vi "Populate Tree Control Recursive Priv.vi"(4 "Show IDs (True)":bool=TRUE, 6 "Indent":i32, 7 "Data Types Dict":variant, 8 "error in":errorcluster, 9 "Items":T1(array[cluster]), 10 "Child IDs":string[](array[string]), 11 "Tree Dictionary In":variant) -> (0 "error out":errorcluster, 1 "Items Out":T1(array[cluster]), 3 "Tree Dictionary Out":variant)   [LabVIEW 2017, in "Tree API.lvlib" / "Tree.lvclass"]
uses:
  Tree.lvclass
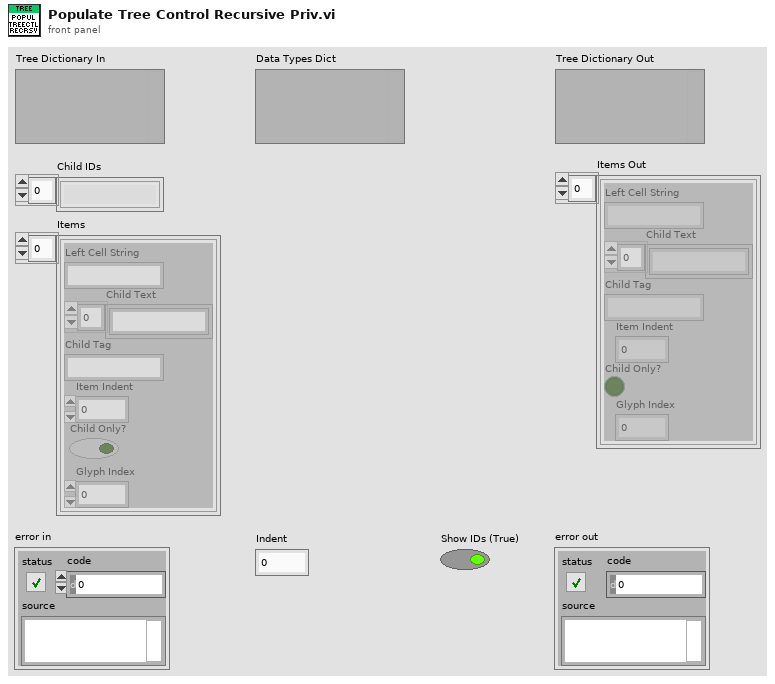
[diagram p1: front panel]
types:
  T1 = cluster{"Left Cell String":string, "Child Text":string[], "Child Tag":string, "Item Indent":i32, "Child Only?":bool, "Glyph Index":i32}[]
  T2 = cluster{"Left Cell String":string, "Child Text":string[], "Child Tag":string, "Item Indent":i32, "Child Only?":bool, "Glyph Index":i32}
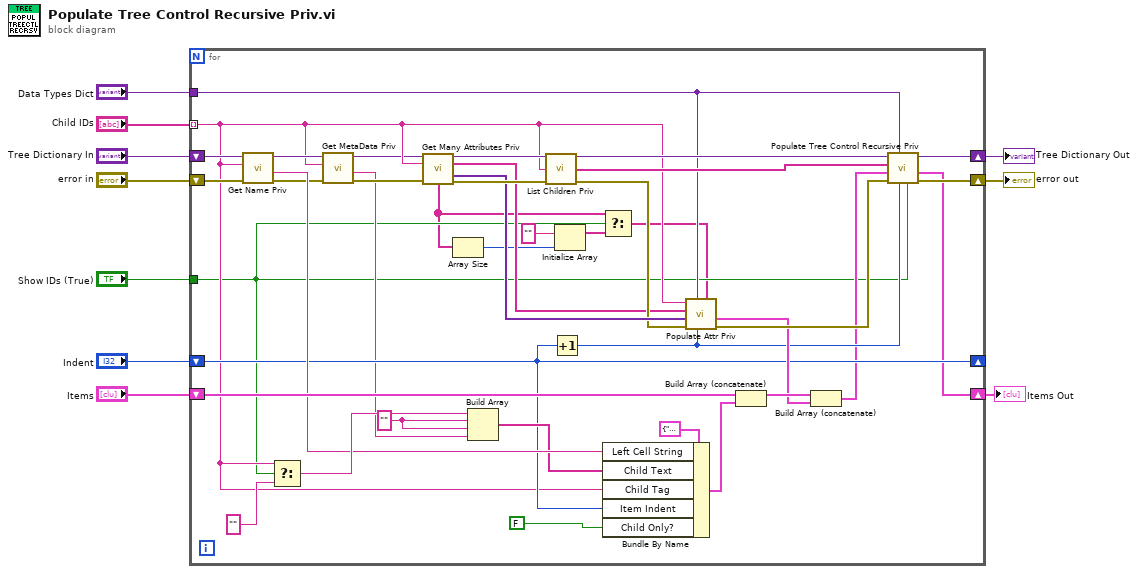
[diagram p0: block diagram]
diagram:
  n1 = for {
    tunnel: "Child IDs" -> [w22] mode=indexing
    shift-right: [w45] -> w7
    shift-left: "Tree Dictionary In" -> [w48]
    shift-right: [w43] -> w10
    shift-left: "error in" -> [w47]
    tunnel: "Show IDs (True)" -> [w16]
    tunnel: "Data Types Dict" -> [w24]
    shift-right: [w25] -> w1
    shift-left: "Items" -> [w36]
    shift-right: [w28] -> _
    shift-left: "Indent" -> [w28]
    w17 = "" ("element")
    n2 = call "Get Name Priv.vi"("error in"=w47, "Unique ID"=w22, "Tree Dictionary"=w48) -> ("error out"=w21:errorcluster, "Name"=w34:string, "Tree Dictionary Out"=w23:variant)  [unwired: 6 in]
    n3 = Select(t=w22, s=w16, f="") -> (s? t:f=w38:string)
    n4 = call "Get MetaData Priv.vi"("error in"=w21, "Unique ID"=w22, "Tree Dictionary"=w23) -> ("error out"=w19:errorcluster, "MetaData"=w18:string, "Tree Dictionary Out"=w20:variant)  [unwired: 6 in]
    n5 = call "Get Many Attributes Priv.vi"("Tree Dictionary In"=w20, "Unique ID"=w22, "error in"=w19) -> ("Tree Dictionary Out"=w50:variant, "Attribute Names"=w37:string[], "Attribute Values"=w41:variant[], "Data IDs"=w13:string[], "error out"=w49:errorcluster)  [unwired: 7 in, 1 out]
    n6 = Array Size(array=w13) -> (size(s)=w15:i32)
    n7 = Build Array(w38, w17, w17, w18) -> (w32:string[])
    n8 = call "List Children Priv.vi"("Tree Dictionary"=w50, "Parent ID"=w22, "Error In"=w49) -> ("Tree Dictionary Out"=w46:variant, "Child IDs"=w44:string[], "Error Out"=w40:errorcluster)  [unwired: 10 in]
    n9 = Increment(x=w28) -> (x+1=w27:i32)
    n10 = Initialize Array("" ("Name"), w15) -> (w12:string[])
    n11 = Select(t=w13, s=w16, f=w12) -> (s? t:f=w11:string[])
    n12 = Bundle By Name(cluster=T2 {"Left Cell String"="", "Child Text"=[], "Child Tag"="", "Item Indent"=0, "Child Only?"=FALSE, "Glyph Index"=0} ("Item"), "Left Cell String"=w34, "Child Text"=w32, "Child Tag"=w22, "Item Indent"=w28, "Child Only?"=FALSE) -> (w31:T2)
    n13 = call "Populate Attr Priv.vi"("Attribute IDs"=w11, "Item Indent"=w27, "Data Types Dict"=w24, "error in"=w40, "Attribute Values"=w41, "Attribute Names"=w37, "Unique ID"=w22) -> ("error out"=w42:errorcluster, "Attr Items"=w29:T1)  [unwired: 3 in]
    n14 = Build Array (concatenate)(w36, w31) -> (w30:T1)
    n15 = Build Array (concatenate)(w30, w29) -> (w26:T1)
    n16 = call "Populate Tree Control Recursive Priv.vi"("Show IDs (True)"=w16, "Indent"=w27, "Data Types Dict"=w24, "error in"=w42, "Items"=w26, "Child IDs"=w44, "Tree Dictionary In"=w46) -> ("error out"=w43:errorcluster, "Items Out"=w25:T1, "Tree Dictionary Out"=w45:variant)  [unwired: 2 in]
  }
  "error out" <- w10
  "Tree Dictionary Out" <- w7
  "Items Out" <- w1
